vi "Harry_Kane_Calibirattion.vi"() -> ()   [LabVIEW 2013]
uses:
  <vilib>/vision/driver/NI_Vision_Acquisition_Software.lvlib
  <vilib>/vision/NI_Vision_Development_Module.lvlib
  <vilib>/vision/Calibration.llb/Distortion Model Types.ctl
  <vilib>/vision/Calibration.llb/Distortion Model.ctl
panel:
  in  "Images Tab":T1(tab)
  out "Image":T2(plugin-control)
  out "Calibration Grid":T2(plugin-control)
  out "Calibration Error Statistics":T3
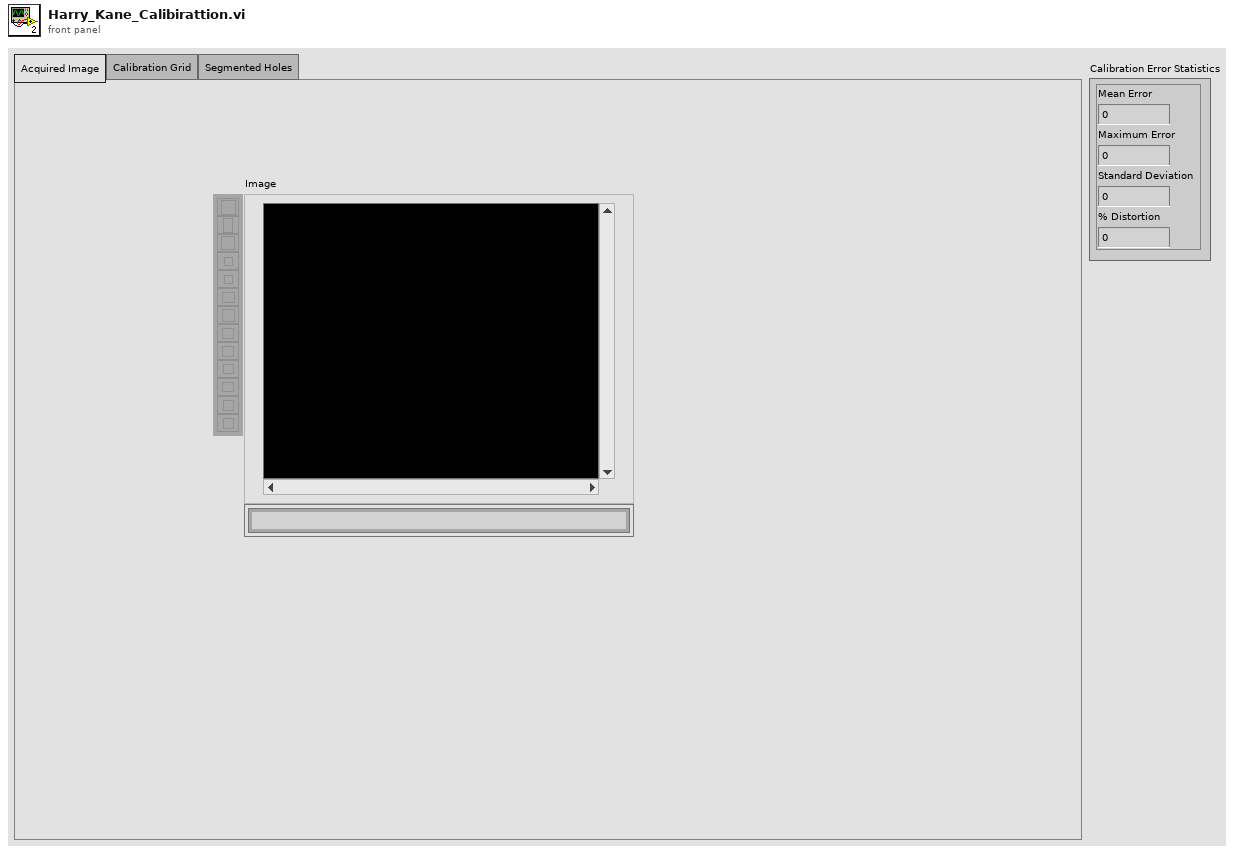
[diagram p1: front panel]
types:
  T1 = enum32{"Acquired Image", "Calibration Grid", "Segmented Holes"}
  T2 = typedef "IMAQ Image.ctl" = refnum<image>
  T3 = cluster{"Mean Error":dbl, "Maximum Error":dbl, "Standard Deviation":dbl, "% Distortion":dbl}
  T4 = typedef "Image Type" = u32
  T5 = typedef "IMAQdx.ctl" = refnum<k21>
  T6 = typedef "Image Unit" = enum32{"Undefined", "Angström", "Micrometer", "Millimeter", "Centimeter", "Meter", "Kilometer", "Microinch", "Inch", "Feet", "Nautical miles", "Standard miles", "Steps"}
  T7 = typedef "Distortion Model.ctl" = cluster{"Distortion Model":T8, "Polynomial Model Setup":cluster{"Radial Coefficient":u32, "Tangential Coefficients ":bool}}
  T8 = typedef "Distortion Model Types.ctl" = i32
  T9 = typedef "Particle Parameters" = i32
  T10 = cluster{"Measurement Parameter":T9, "Range Lower Value":dbl, "Range Upper Value":dbl, "Range":bool, "Measurement Type":bool}[]
  T11 = typedef "Calibration Reference Points.ctl" = cluster{"Pixel Coordinates":cluster{"X":dbl, "Y":dbl}[], "Real World Coordinates":cluster{"X":dbl, "Y":dbl}[], "Unit":T6, "Image Size":cluster{"X":u32, "Y":u32}}
  T12 = typedef "Error Statistics.ctl" = cluster{"Mean Error":dbl, "Maximum Error":dbl, "Standard Deviation":dbl, "% Distortion":dbl}
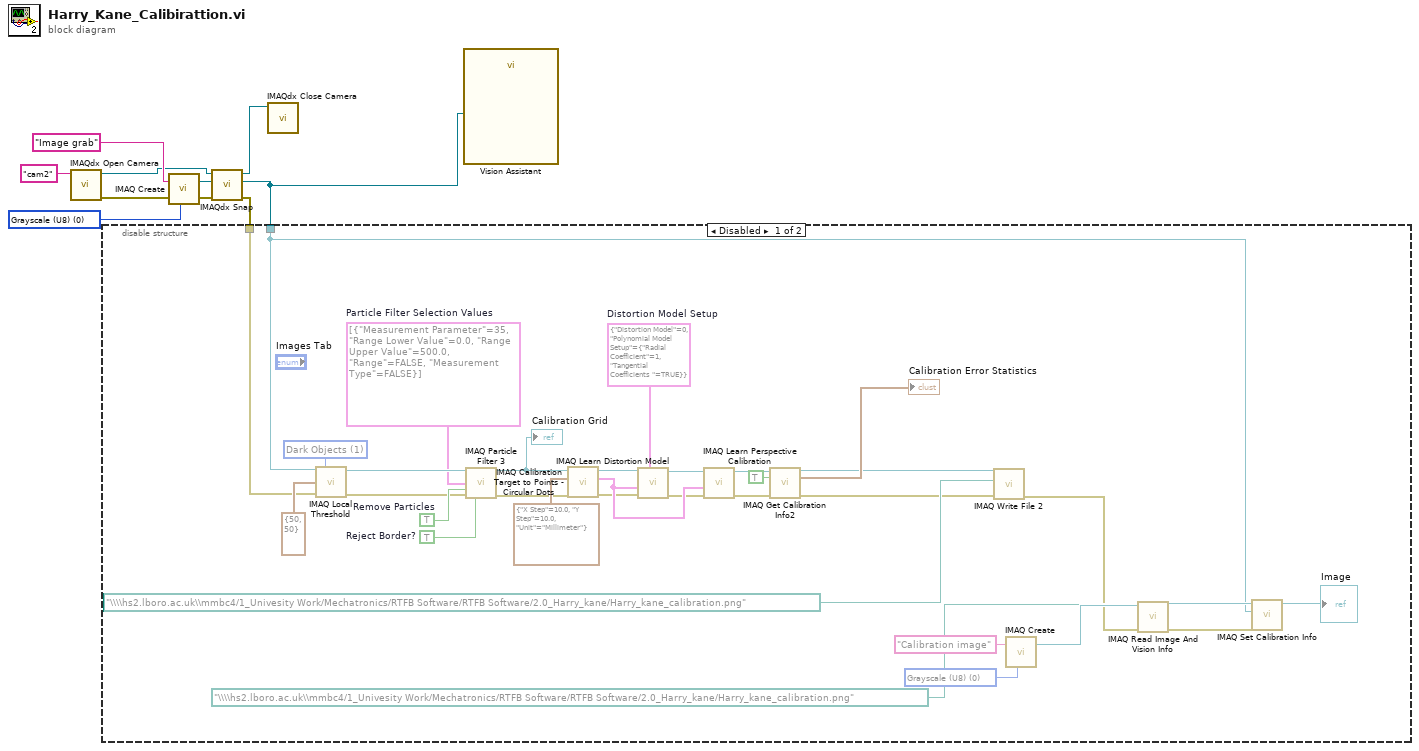
[diagram p0: block diagram]
diagram:
  w9 = T4 0 items=["Grayscale (U8)", "Grayscale (I16)", "Grayscale (SGL)", "Complex (CSG)", "RGB (U32)", "HSL (U32)", "RGB (U64)", "Grayscale (U16)"] ("Image Type")
  n1 = call <vilib>:"IMAQdx Open Camera.vi"("Session In"="cam2" ("Interface Name")) -> ("error out"=w4:errorcluster, "Session Out"=w5:T5)  [unwired: 9 in]
  n2 = call "IMAQ Create"("Image Name"="Image grab", "Image Type"=w9, "error in (no error)"=w4) -> ("New Image"=w8:T2, "error out"=w7:errorcluster)  [unwired: 2 in]
  n3 = call <vilib>:"IMAQdx Snap.vi"("error in"=w7, "Image In"=w8, "Session In"=w5) -> ("error out"=w2:errorcluster, "Image Out"=w1:T2, "Session Out"=w3:T5)  [unwired: 6 in]
  n4 = disable-structure shown="Disabled" {
    disable-tunnel: w2 -> [w23 _]
    disable-tunnel: w1 -> [w15 _]
    frame Disabled {
      w12 = T4 0 items=["Grayscale (U8)", "Grayscale (I16)", "Grayscale (SGL)", "Complex (CSG)", "RGB (U32)", "HSL (U32)", "RGB (U64)", "Grayscale (U16)"] ("Image Type")
      w30 = T7 {"Distortion Model"=0, "Polynomial Model Setup"={"Radial Coefficient"=1, "Tangential Coefficients "=TRUE}}  # Distortion Model Setup
      w31 = T10 [{"Measurement Parameter"=35, "Range Lower Value"=0.0, "Range Upper Value"=500.0, "Range"=FALSE, "Measurement Type"=FALSE}]  # Particle Filter Selection Values
      w34 = TRUE  # Remove Particles
      w33 = TRUE  # Reject Border?
      w42 = u32 1 items=["Bright Objects", "Dark Objects"] ("Look For (Bright Objects)")
      n5 = call "IMAQ Local Threshold"("Image Src"=w15, "Look For (Bright Objects)"=w42, "Window Size (32x32)"=cluster{"SizeX":i32, "SizeY":i32} {"SizeX"=50, "SizeY"=50}, "error in (no error)"=w23) -> ("Image Dst Out"=w32:T2, "error out"=w29:errorcluster)  [unwired: 4 in, 6 out]
      n6 = call "IMAQ Particle Filter 3"("Image Src"=w32, "Selection Values"=w31, "Keep/Remove Particles (F)"=w34, "error in (no error)"=w29, "Reject Border? (F)"=w33) -> ("Image Dst Out"=w24:T2, "error out"=w28:errorcluster)  [unwired: 4 in, 5 out]
      "Calibration Grid" <- w24
      n7 = call "IMAQ Calibration Target to Points - Circular Dots"("error in (no error)"=w28, "Grid Descriptor"=cluster{"X Step":sgl, "Y Step":sgl, "Unit":T6} {"X Step"=10.0, "Y Step"=10.0, "Unit"=enum."Millimeter"}, "Target Image"=w24) -> ("error out"=w27:errorcluster, "Reference Points"=w39:T11, "Target Image (dup)"=w41:T2)  [unwired: 2 in, 4 out]
      n8 = call "IMAQ Learn Distortion Model"("Distortion Model Setup"=w30, "error in (no error)"=w27, "Reference Points"=w39, "Calibration Template Image"=w41) -> ("error out"=w26:errorcluster, "Calibration Template Image Out"=w40:T2)  [unwired: 2 in, 4 out]
      n9 = call "IMAQ Learn Perspective Calibration"("error in (no error)"=w26, "Reference Points"=w39, "Calibration Template Image"=w40) -> ("error out"=w25:errorcluster, "Calibration Template Image Out"=w38:T2)  [unwired: 1 in, 6 out]
      n10 = call "IMAQ Get Calibration Info2"("Calibration Template Image"=w38, "Return Error Information (False)"=TRUE, "error in (no error)"=w25) -> ("Calibration Template Image (duplicate)"=w22:T2, "Error Statistics"=→"Calibration Error Statistics":T12, "error out"=w20:errorcluster)  [unwired: 10 out]
      n11 = call-poly "IMAQ Write File 2"("error in (no error)"=w20, "File Path"=path "\\\\hs2.lboro.ac.uk\\mmbc4/1_Univesity Work/Mechatronics/RTFB Software/RTFB Software/2.0_Harry_kane/Harry_kane_calibration.png", "Image"=w22) -> ("error out"=w17:errorcluster)  [unwired: 7 in, 1 out]
      n12 = call "IMAQ Create"("Image Name"="Calibration image", "Image Type"=w12) -> ("New Image"=w19:T2)  [unwired: 3 in, 1 out]
      n13 = call "IMAQ Read Image And Vision Info"("File Path"=path "\\\\hs2.lboro.ac.uk\\mmbc4/1_Univesity Work/Mechatronics/RTFB Software/RTFB Software/2.0_Harry_kane/Harry_kane_calibration.png", "error in (no error)"=w17, "Image"=w19) -> ("error out"=w13:errorcluster, "Image Out"=w16:T2)  [unwired: 6 in, 1 out]
      n14 = call "IMAQ Set Calibration Info"("error in (no error)"=w13, "Image Dst"=w15, "Image Src"=w16) -> ("Calibrated Image"=→"Image":T2)  [unwired: 7 in, 1 out]
    }
    frame Enabled {
    }
  }
  n15 = call <vilib>:"IMAQdx Close Camera.vi"("Session In"=w3) -> ()  [unwired: 10 in, 1 out]
  n16 = call "Vision Assistant"("Image In"=w1) -> ()  [unwired: 25 in, 2 out]
